vi "Reset.vi"(8 "ErrorArray In":errorcluster[](array[cluster]), 11 "NISTBus In":refnum<class "NISTBus.lvclass">) -> (0 "ErrorArray Out":errorcluster[](array[cluster]), 3 "NISTBus Out":refnum<class "NISTBus.lvclass">)   [LabVIEW 2014, in "Bus.lvlib" / "NISTBus.lvclass"]
uses:
  NISTBus.lvclass
  <userlib>/NIST/NISTErrorLib/NISTErrorLib.lvlib
  FGenPlugins/MyPluginBaseClass/NISTFGenPluginsBase.lvclass
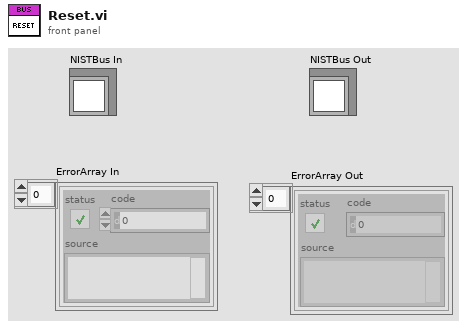
[diagram p1: front panel]
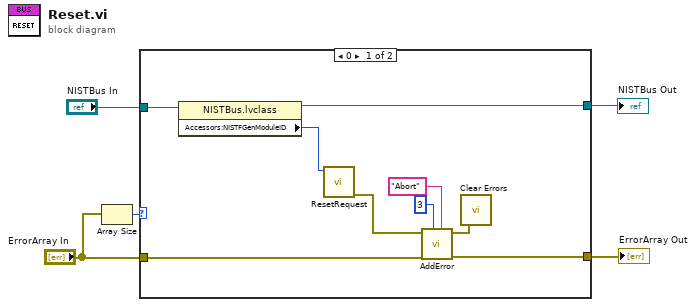
[diagram p0: block diagram]
diagram:
  n1 = Array Size(array="ErrorArray In") -> (size(s)=w5:i32)
  n2 = case shown="0" w5 {
    tunnel: "ErrorArray In" -> [w11 w16]
    tunnel: [w10 w16] -> w3
    tunnel: "NISTBus In" -> [w9 w15]
    tunnel: [w8 w15] -> w1
    frame 0 {
      n3 = property class="NISTBus.lvclass"(reference=w9) -> (reference out=w8:refnum<class "NISTBus.lvclass">, "Accessors:NISTFGenModuleID"=w6:i32)  [unwired: 1 in, 1 out]
      n4 = call "ResetRequest.vi"("ModuleID"=w6) -> ("error out"=w7:errorcluster)  [unwired: 10 in]
      n5 = call <userlib>:"AddError.vi"("Severity"="Abort" ("String"), "Priority"=u8 3, "ErrorArray"=w11, "error in (no error)"=w7) -> ("ErrorArray"=w10:errorcluster[], "error out"=w12:errorcluster)  [unwired: 6 in]
      n6 = call <vilib>:"Clear Errors.vi"("error in (no error)"=w12) -> ()  [unwired: 5 in, 2 out]
    }
    frame 1, Default {
    }
  }
  "NISTBus Out" <- w1
  "ErrorArray Out" <- w3
